vi "crio_FPGA_Antagonist_Radial.vi"() -> ()   [LabVIEW 2019]
uses:
  <vilib>/rvi/Analysis/control/PID/Typedef/niFpgaPID_ManualControl.ctl
  <vilib>/rvi/Analysis/control/PID/Typedef/niFpgaPID_PIGains.ctl
  <vilib>/rvi/Analysis/control/PID/Typedef/niFpgaPID_OutputRange.ctl
  <vilib>/rvi/Emulation/niFpgaSctlEmulationGetInTimedLoop.vi
  <vilib>/rvi/Emulation/niFpgaProcessEmulError.vi
  <vilib>/rvi/eio/common/nirviEmuTemplateMethod_errors.vi
  <vilib>/rvi/Emulation/niFpgaGetClockAttributes.vi
  <vilib>/rvi/Emulation/niFpgaEmulationReportErrorSimple.vi
  <vilib>/rvi/Emulation/niFpgaCriticalErrorInLSC.vi
  <vilib>/rvi/Analysis/control/PID/SubVIs/niFpgaPID_PIWrapper.vi
  <vilib>/eio/EIOMethodNode/EIOMethodNode.xnode
  <vilib>/eio/EIONode/EIONode.xnode
panel:
  in  "LAC Lock":bool
  in  "VCA Gains":T1 {"proportional gain" step=0.125}
  in  "LAC DC PWM Period (us)":i16=50
  in  "Debug: ConnectorA/DIO15":bool
  in  "Debug: ConnectorA/DIO14":bool
  in  "Encoder Debug":bool
  in  "Loop Timer DAQ":u32=1 caption="LAC Loop Time(uSec)"
  in  "Position Reset":bool
  out "LAC Position (Counts)":i32
  out "LAC B":bool
  out "LAC A":bool
  out "LAC B'":bool
  out "LAC A'":bool
  in  "LAC Velocity Interval (uSec)":u32=1000
  out "LAC Acceleration (Counts/Interval)":i32
  out "LAC Velocity (Counts/Interval)":i32
  out "LAC Controller PWM Output":sgl
  in  "LAC Manual Control":T2 {"manual input (0)" scale=-1.0..1.0}
  in  "LAC Setpoint":i32
  in  "LAC Gains":T1 {"proportional gain" step=0.125}
  in  "stop 2":bool
  in  "rail Initial Position":i16=1
  out "rail Platform Position":i16
  in  "Stepper Direction":bool
  in  "Stepper Enable":bool
  in  "Position Control: Desired Positoin":i16=100
  in  "Manual Operation":bool
  out "Controller Enable":bool
  out "Controller Direction":bool
  in  "mSec to initialize a small push away from limit switch":u32=1 caption="mSec when hit limit"
  in  "mSec when hit limit":u32=100 caption="rail mSec to pause when hit limit"
  in  "Rail soft limit":i16=10000
  out "Limit Switch":bool
  in  "Half Peirod (pulse 40MHz)":u32=10000 caption="rail Count(Tick) [Interval between step]"
  out "VCA ControllerPWM Output":sgl
  in  "VCA Manual Control":T2 {"manual input (0)" scale=-1.0..1.0}
  in  "VCA Position Setpoint":i32
  in  "Loop Timer DAQ 2":u32=1 caption="Loop Time(uSec)"
  in  "VCA Position Reset":bool
  out "Position (Counts) VCA":i32=-5
  out "B VCA":bool
  out "A VCA":bool=TRUE
  out "B' VCA":bool
  out "A' VCA":bool=TRUE
  in  "Velocity Interval (uSec)":u32=1000
  out "Acceleration (Counts/Interval) VCA":i32
  out "Velocity (Counts/Interval) VCA":i32
  in  "DC PWM Period (microsec)":i16=50
  in  "stop":bool=TRUE
  # "Period Default 500(us) 2kHz"
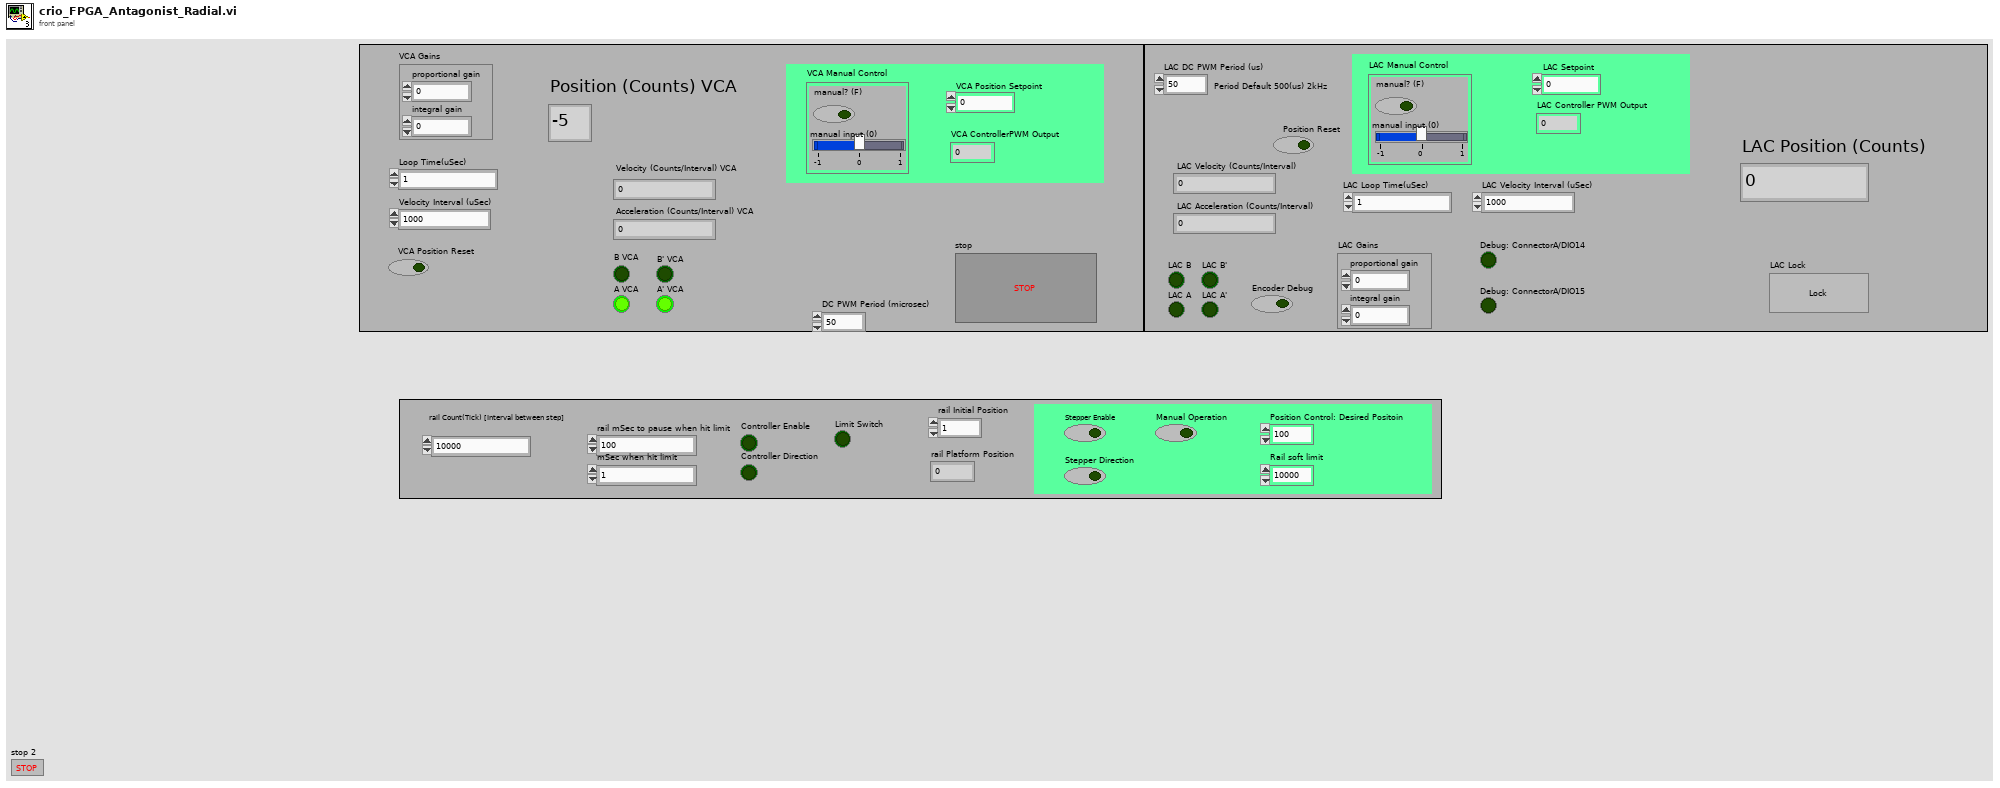
[diagram p1: front panel]
types:
  T1 = typedef "niFpgaPID_PIGains.ctl" = cluster{"proportional gain":sgl, "integral gain":sgl}
  T2 = typedef "niFpgaPID_ManualControl.ctl" = cluster{"manual? (F)":bool, "manual input (0)":sgl}
  T3 = typedef "niFpgaPID_OutputRange.ctl" = cluster{"output high (Inf)":sgl, "output low (-Inf)":sgl}
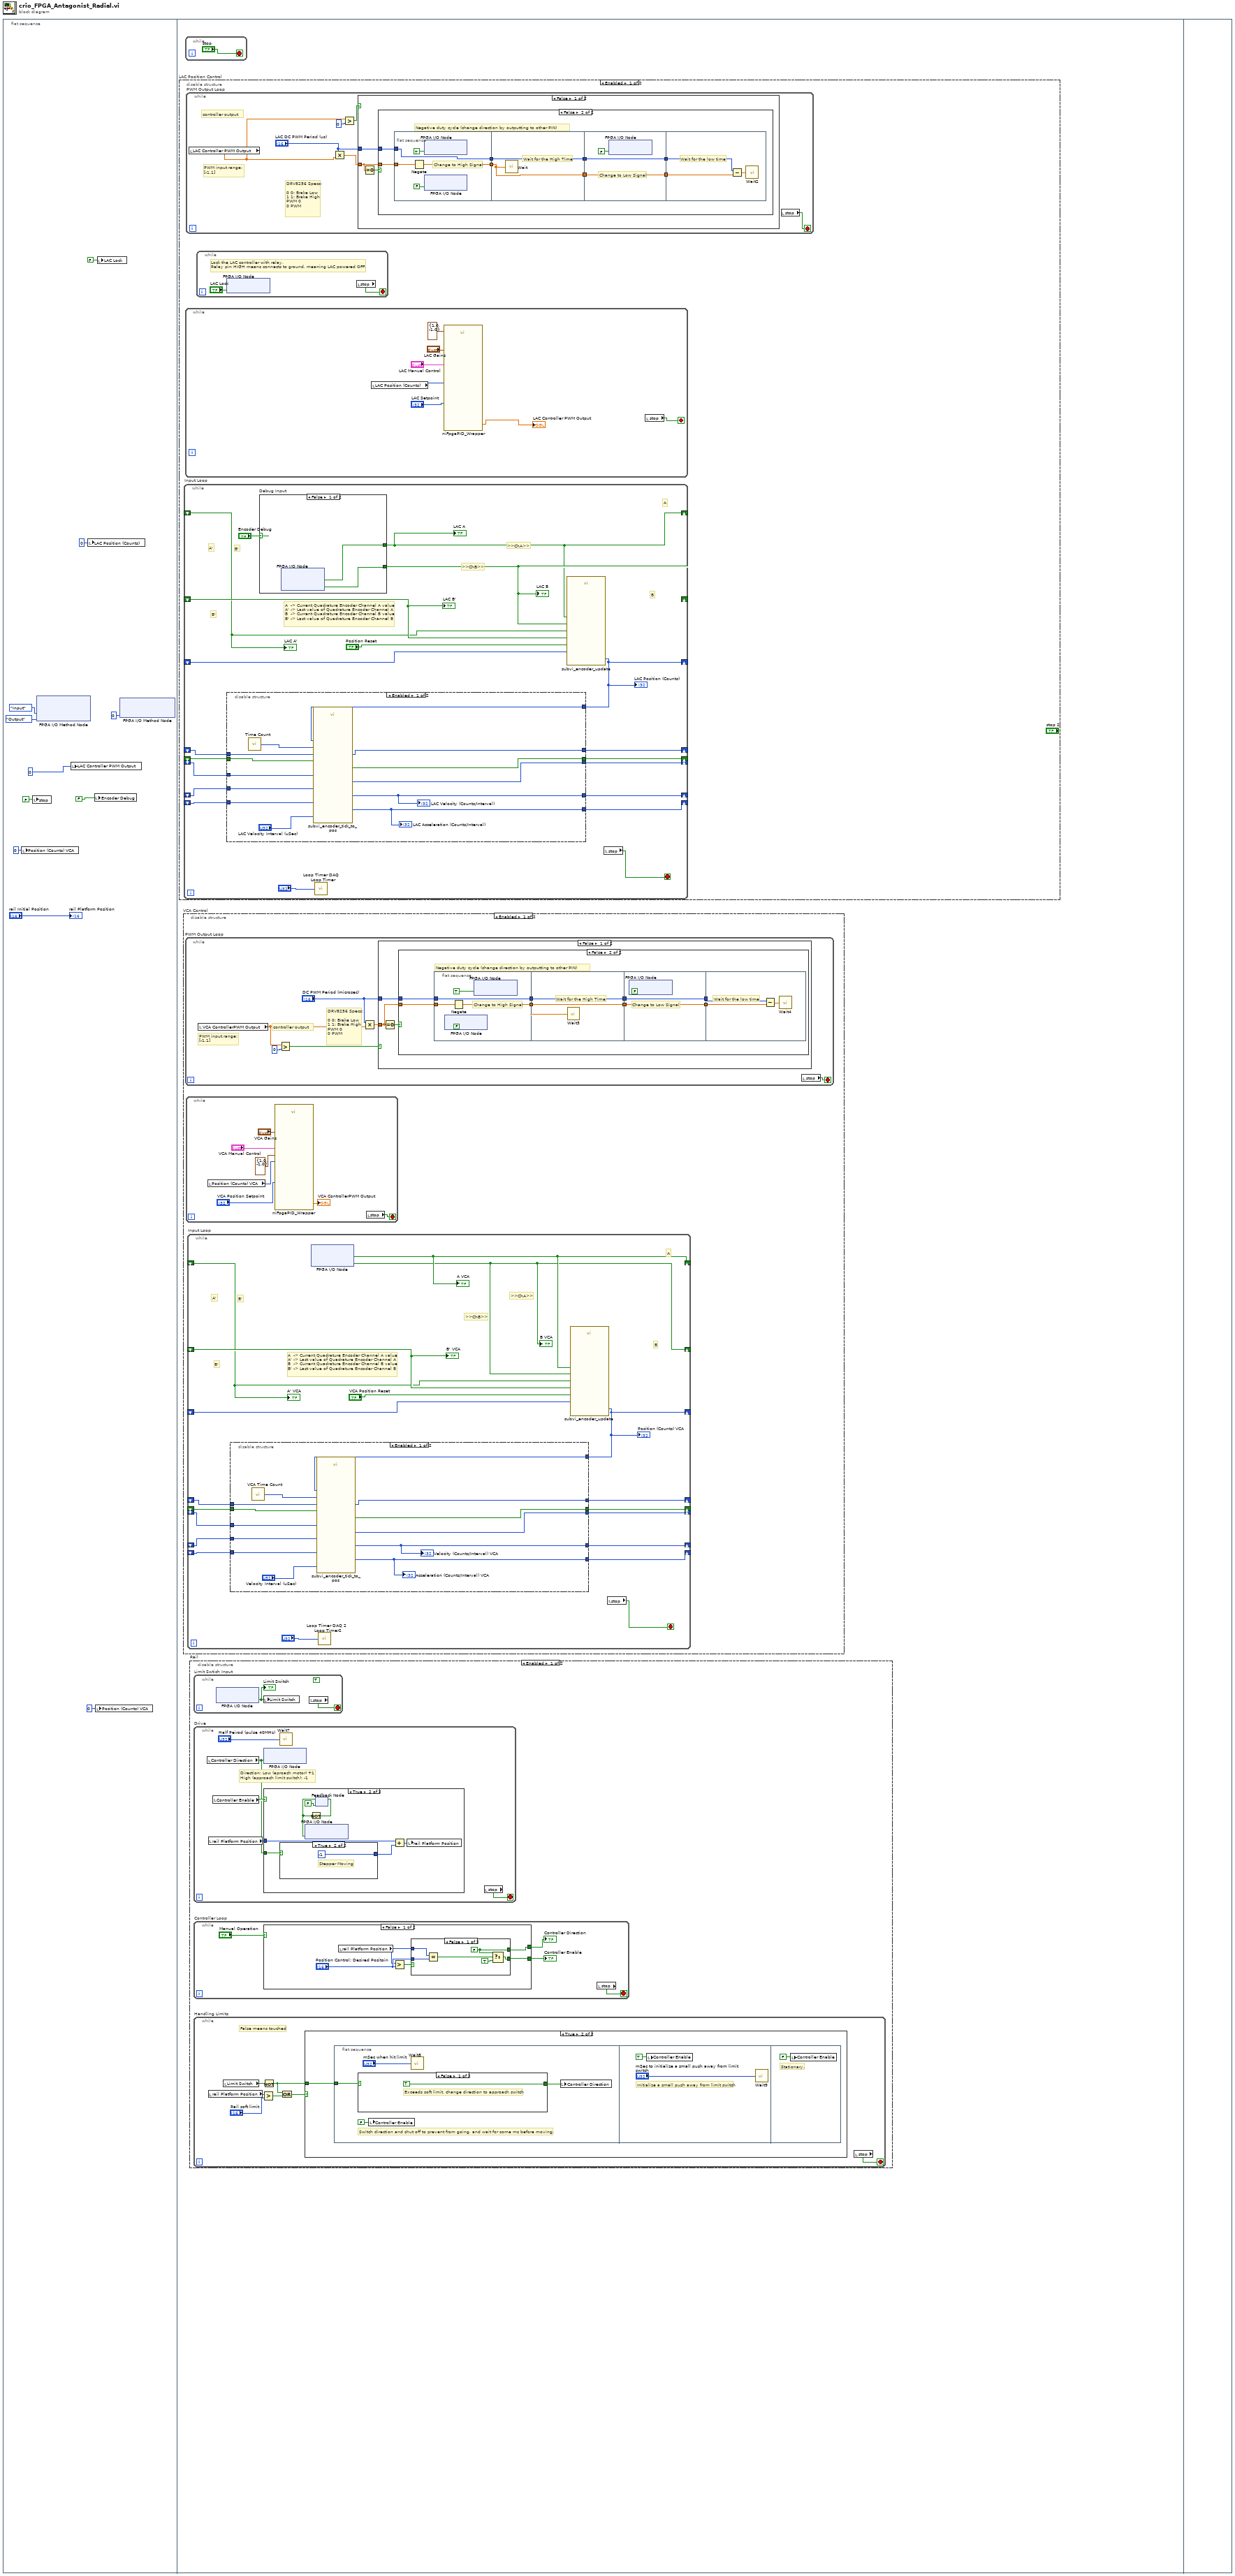
[diagram p0: block diagram]
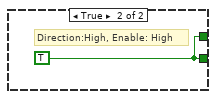
[diagram p2: hidden frame]
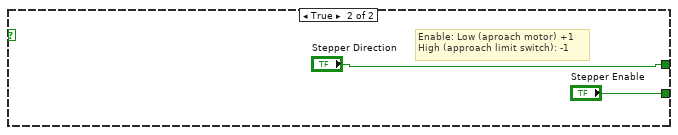
[diagram p3: hidden frame]
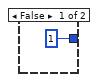
[diagram p5: hidden frame]
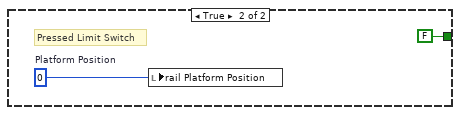
[diagram p7: hidden frame]
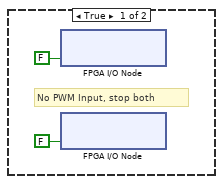
[diagram p10: hidden frame]
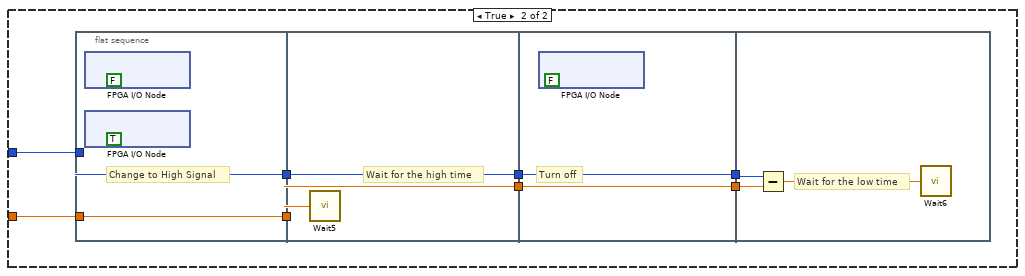
[diagram p11: hidden frame]
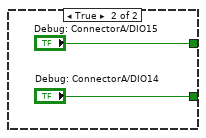
[diagram p14: hidden frame]
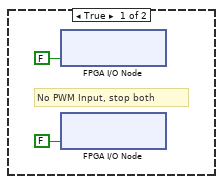
[diagram p15: hidden frame]
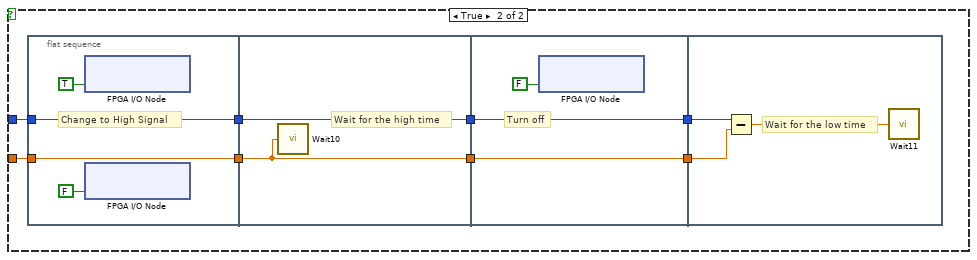
[diagram p16: hidden frame]
diagram:
  n1 = flat-sequence {
    frame #0 {
      n2 = local write "Position (Counts) VCA"(0 ("LAC Position (Counts)")) -> ()
      n3 = local write "stop"(FALSE ("stop")) -> ()
      n4 = xnode "FPGA I/O Method Node"("DIO 7:4"=enum8{"No Change", "Input", "Output"}."Input", "DIO 3:0"=enum8{"No Change", "Input", "Output"}."Output") -> ()  [unwired: 1 in, 1 out]
      n5 = local write "LAC Controller PWM Output"(u32 0 ("Servo wait time")) -> ()
      n6 = local write "LAC Position (Counts)"(0 ("LAC Position (Counts)")) -> ()
      n7 = local write "Encoder Debug"(FALSE ("LAC Lock")) -> ()
      n8 = local write "Position (Counts) VCA"(0 ("Position (Counts) VCA")) -> ()
      n9 = local write "LAC Lock"(FALSE ("LAC Lock")) -> ()
      n10 = xnode "FPGA I/O Method Node"("Enable"=u8 0) -> ()  [unwired: 1 in, 1 out]
      "rail Platform Position" <- "rail Initial Position"
    }
    frame #1 {
      n11 = disable-structure "LAC Position Control" shown="Enabled" {
        frame Enabled {
          n12 = while "Input Loop" {
            shift-right: [w178] -> _
            shift-left: _ -> [w181]
            shift-right: [w177] -> _
            shift-left: _ -> [w180]
            shift-right: [w173] -> _
            shift-left: _ -> [w179]
            shift-right: [w166] -> _
            shift-left: _ -> [w176]
            shift-right: [w167] -> _
            shift-left: _ -> [w175]
            shift-right: [w174] -> _
            shift-left: _ -> [w172]
            shift-right: [w171] -> _
            shift-left: _ -> [w170]
            shift-right: [w169] -> _
            shift-left: _ -> [w168]
            stop <- w165 stop-if-true
            # "B'"
            # ">>ChB>>"
            # ">>ChA>>"
            # "A'"
            # "A  -> Current Quadrature Encoder Channel A value\nA' -> Last value of Quadrature Encoder Channel A\nB  -> Current Quadrature Encoder Channel B value\nB' -> Last value of Quadrature Encoder Channel B"
            # "B'"
            # "B"
            # "A"
            n13 = case "Debug Input" shown="False" "Encoder Debug" {
              tunnel: [w199 "Debug: ConnectorA/DIO15"] -> w177
              tunnel: [w198 "Debug: ConnectorA/DIO14"] -> w178
              frame False {
                n14 = xnode "FPGA I/O Node"() -> ("Mod2/DIO2"=w199:bool, "Mod2/DIO3"=w198:bool)  [unwired: 2 in, 2 out]
              }
              frame True {
              }
            }
            "LAC B" <- w178
            "LAC A" <- w177
            n15 = call "Loop Timer"("Count(uSec)"="Loop Timer DAQ") -> ()  [unwired: 1 out]
            n16 = call "subvi_encoder_update.vi"("Position Reset"="Position Reset", "Tick'"=w179, "A"=w177, "B'"=w181, "A'"=w180, "B"=w178) -> ("Tick"=w173:i32)  [unwired: 5 in]
            "LAC Position (Counts)" <- w173
            n17 = disable-structure shown="Enabled" {
              disable-tunnel: w176 -> [w196 _]
              disable-tunnel: w175 -> [w195 _]
              disable-tunnel: [w194 _] -> w174
              disable-tunnel: w173 -> [w193 _]
              disable-tunnel: w172 -> [w192 _]
              disable-tunnel: [w191 _] -> w171
              disable-tunnel: w170 -> [w190 _]
              disable-tunnel: [w189 _] -> w169
              disable-tunnel: w168 -> [w188 _]
              disable-tunnel: [w186 _] -> w167
              disable-tunnel: [w185 _] -> w166
              frame Enabled {
                n18 = call "Time Count"() -> ("Tick Count(uSec)"=w187:u32)
                n19 = call "subvi_encoder_tick_to_pos.vi"("Velocity Interval (uSec)"="LAC Velocity Interval (uSec)", "Raw Tick"=w193, "Waited?'"=w190, "Tick Count(uSec)'"=w188, "p'"=w192, "Time Count"=w187, "a'"=w195, "v'"=w196) -> ("Waited?"=w191:bool, "Tick Count(uSec)"=w189:u32, "p"=w194:i32, "a"=w186:i32, "v"=w185:i32)  [unwired: 3 in]
                "LAC Acceleration (Counts/Interval)" <- w186
                "LAC Velocity (Counts/Interval)" <- w185
              }
              frame Disabled {
              }
            }
            n20 = local read "stop"() -> (w165:bool)
            "LAC B'" <- w181
            "LAC A'" <- w180
          }
          n21 = while {
            stop <- w164 stop-if-true
            n22 = local read "LAC Position (Counts)"() -> (w163:i32)
            n23 = call-poly <vilib>:"niFpgaPID_Wrapper.vi"("setpoint"="LAC Setpoint", "process variable"=w163, "manual control"="LAC Manual Control", "gains"="LAC Gains", "output range"=T3 {"output high (Inf)"=1.0, "output low (-Inf)"=-1.0}) -> ("output"=→"LAC Controller PWM Output":sgl)  [unwired: 8 in, 2 out]
            n24 = local read "stop"() -> (w164:bool)
          }
          n25 = while "PWM Output Loop" {
            stop <- w202 stop-if-true
            # "PWM input range:\n[-1,1]"
            # "DRV8256 Specs:\n\n0 0: Brake Low\n1 1: Brake High\nPWM 0\n0 PWM"
            # "controller output"
            n26 = local read "LAC Controller PWM Output"() -> (w203:sgl)
            n27 = Multiply(x="LAC DC PWM Period (us)", y=w203) -> (x*y=w205:sgl)
            n28 = Greater?(x=w203, y=i16 0) -> (0:w206:bool)
            n29 = case shown="False" w206 {
              tunnel: w205 -> [w210 w241]
              tunnel: "LAC DC PWM Period (us)" -> [w208 w240]
              frame False {
                n30 = Equal To 0?(x=w210) -> (x = 0?=w209:bool)
                n31 = case shown="False" w209 {
                  tunnel: w210 -> [_ w220]
                  tunnel: w208 -> [_ w213]
                  frame True {
                    # "No PWM Input, stop both"
                    n32 = xnode "FPGA I/O Node"("Mod1/DIO2"=FALSE) -> ()  [unwired: 1 in, 1 out]
                    n33 = xnode "FPGA I/O Node"("Mod1/DIO3"=FALSE) -> ()  [unwired: 1 in, 1 out]
                  }
                  frame False {
                    # "Negative duty cycle (change direction by outputting to other PIN)"
                    n34 = flat-sequence {
                      tunnel: w220 -> [w223]
                      tunnel: [w222] -> w219
                      tunnel: [w221] -> w214
                      tunnel: w213 -> [w221]
                      tunnel: w219 -> [w227]
                      tunnel: [w227] -> w218
                      tunnel: [w226] -> w215
                      tunnel: w214 -> [w226]
                      tunnel: w218 -> [w229]
                      tunnel: [w229] -> w217
                      tunnel: [w228] -> w216
                      tunnel: w215 -> [w228]
                      tunnel: w217 -> [w233]
                      tunnel: w216 -> [w232]
                      frame #0 {
                        # "Change to High Signal"
                        n35 = Negate(x=w223) -> (-x=w222:sgl)
                        n36 = xnode "FPGA I/O Node"("Mod1/DIO3"=TRUE) -> ()  [unwired: 1 in, 1 out]
                        n37 = xnode "FPGA I/O Node"("Mod1/DIO2"=FALSE) -> ()  [unwired: 1 in, 1 out]
                      }
                      frame #1 {
                        # "Wait for the High Time"
                        n38 = call "Wait"("Count(uSec)"=w227) -> ()  [unwired: 1 out]
                      }
                      frame #2 {
                        # "Change to Low Signal"
                        n39 = xnode "FPGA I/O Node"("Mod1/DIO2"=FALSE) -> ()  [unwired: 1 in, 1 out]
                      }
                      frame #3 {
                        # "Wait for the low time"
                        n40 = Subtract(x=w232, y=w233) -> (x-y=w231:sgl)
                        n41 = call "Wait2"("Count(uSec)"=w231) -> ()  [unwired: 1 out]
                      }
                    }
                  }
                }
              }
              frame True {
                n42 = flat-sequence {
                  tunnel: w241 -> [w242]
                  tunnel: w240 -> [w243]
                  tunnel: [w243] -> w237
                  tunnel: [w242] -> w236
                  tunnel: [w247] -> w238
                  tunnel: w237 -> [w247]
                  tunnel: w236 -> [w246]
                  tunnel: [w246] -> w235
                  tunnel: [w249] -> w239
                  tunnel: w238 -> [w249]
                  tunnel: w235 -> [w248]
                  tunnel: [w248] -> w234
                  tunnel: w239 -> [w253]
                  tunnel: w234 -> [w251]
                  frame #0 {
                    # "Change to High Signal"
                    n43 = xnode "FPGA I/O Node"("Mod1/DIO2"=TRUE) -> ()  [unwired: 1 in, 1 out]
                    n44 = xnode "FPGA I/O Node"("Mod1/DIO3"=FALSE ("ConnectorB/DIO9")) -> ()  [unwired: 1 in, 1 out]
                  }
                  frame #1 {
                    # "Wait for the high time"
                    n45 = call "Wait10"("Count(uSec)"=w246) -> ()  [unwired: 1 out]
                  }
                  frame #2 {
                    # "Turn off"
                    n46 = xnode "FPGA I/O Node"("Mod1/DIO2"=FALSE) -> ()  [unwired: 1 in, 1 out]
                  }
                  frame #3 {
                    # "Wait for the low time"
                    n47 = Subtract(x=w253, y=w251) -> (x-y=w252:sgl)
                    n48 = call "Wait11"("Count(uSec)"=w252) -> ()  [unwired: 1 out]
                  }
                }
              }
            }
            n49 = local read "stop"() -> (w202:bool)
          }
          n50 = while {
            stop <- w157 stop-if-true
            # "Lock the LAC controller with relay.\nRelay pin HIGH means connects to ground, meaning LAC powered OFF."
            n51 = xnode "FPGA I/O Node"("Mod8/DIO6"="LAC Lock") -> ()  [unwired: 1 in, 1 out]
            n52 = local read "stop"() -> (w157:bool)
          }
        }
        frame Disabled {
        }
      }
      n53 = disable-structure "VCA Control" shown="Enabled" {
        frame Enabled {
          n54 = while "PWM Output Loop" {
            stop <- w104 stop-if-true
            # "PWM input range:\n[-1,1]"
            # "DRV8256 Specs:\n\n0 0: Brake Low\n1 1: Brake High\nPWM 0\n0 PWM"
            # "controller output"
            n55 = local read "VCA ControllerPWM Output"() -> (w105:sgl)
            n56 = Greater?(x=w105, y=i16 0) -> (0:w108:bool)
            n57 = Multiply(x="DC PWM Period (microsec)", y=w105) -> (x*y=w107:sgl)
            n58 = case shown="False" w108 {
              tunnel: w107 -> [w112 w143]
              tunnel: "DC PWM Period (microsec)" -> [w110 w142]
              frame False {
                n59 = Equal To 0?(x=w112) -> (x = 0?=w111:bool)
                n60 = case shown="False" w111 {
                  tunnel: w112 -> [_ w122]
                  tunnel: w110 -> [_ w115]
                  frame True {
                    # "No PWM Input, stop both"
                    n61 = xnode "FPGA I/O Node"("Mod1/DIO1"=FALSE) -> ()  [unwired: 1 in, 1 out]
                    n62 = xnode "FPGA I/O Node"("Mod1/DIO0"=FALSE) -> ()  [unwired: 1 in, 1 out]
                  }
                  frame False {
                    # "Negative duty cycle (change direction by outputting to other PIN)"
                    n63 = flat-sequence {
                      tunnel: w122 -> [w125]
                      tunnel: [w124] -> w121
                      tunnel: [w123] -> w116
                      tunnel: w115 -> [w123]
                      tunnel: w121 -> [w129]
                      tunnel: [w129] -> w120
                      tunnel: [w128] -> w117
                      tunnel: w116 -> [w128]
                      tunnel: w120 -> [w131]
                      tunnel: [w131] -> w119
                      tunnel: [w130] -> w118
                      tunnel: w117 -> [w130]
                      tunnel: w119 -> [w135]
                      tunnel: w118 -> [w134]
                      frame #0 {
                        # "Change to High Signal"
                        n64 = xnode "FPGA I/O Node"("Mod1/DIO0"=FALSE) -> ()  [unwired: 1 in, 1 out]
                        n65 = Negate(x=w125) -> (-x=w124:sgl)
                        n66 = xnode "FPGA I/O Node"("Mod1/DIO1"=TRUE) -> ()  [unwired: 1 in, 1 out]
                      }
                      frame #1 {
                        # "Wait for the High Time"
                        n67 = call "Wait3"("Count(uSec)"=w129) -> ()  [unwired: 1 out]
                      }
                      frame #2 {
                        # "Change to Low Signal"
                        n68 = xnode "FPGA I/O Node"("Mod1/DIO1"=FALSE) -> ()  [unwired: 1 in, 1 out]
                      }
                      frame #3 {
                        # "Wait for the low time"
                        n69 = Subtract(x=w134, y=w135) -> (x-y=w133:sgl)
                        n70 = call "Wait4"("Count(uSec)"=w133) -> ()  [unwired: 1 out]
                      }
                    }
                  }
                }
              }
              frame True {
                n71 = flat-sequence {
                  tunnel: w143 -> [w144]
                  tunnel: w142 -> [w145]
                  tunnel: [w145] -> w139
                  tunnel: [w144] -> w138
                  tunnel: [w149] -> w140
                  tunnel: w139 -> [w149]
                  tunnel: w138 -> [w148]
                  tunnel: [w148] -> w137
                  tunnel: [w151] -> w141
                  tunnel: w140 -> [w151]
                  tunnel: w137 -> [w150]
                  tunnel: [w150] -> w136
                  tunnel: w141 -> [w155]
                  tunnel: w136 -> [w153]
                  frame #0 {
                    # "Change to High Signal"
                    n72 = xnode "FPGA I/O Node"("Mod1/DIO1"=FALSE ("ConnectorB/DIO9")) -> ()  [unwired: 1 in, 1 out]
                    n73 = xnode "FPGA I/O Node"("Mod1/DIO0"=TRUE) -> ()  [unwired: 1 in, 1 out]
                  }
                  frame #1 {
                    # "Wait for the high time"
                    n74 = call "Wait5"("Count(uSec)"=w148) -> ()  [unwired: 1 out]
                  }
                  frame #2 {
                    # "Turn off"
                    n75 = xnode "FPGA I/O Node"("Mod1/DIO0"=FALSE) -> ()  [unwired: 1 in, 1 out]
                  }
                  frame #3 {
                    # "Wait for the low time"
                    n76 = Subtract(x=w155, y=w153) -> (x-y=w154:sgl)
                    n77 = call "Wait6"("Count(uSec)"=w154) -> ()  [unwired: 1 out]
                  }
                }
              }
            }
            n78 = local read "stop"() -> (w104:bool)
          }
          n79 = while {
            stop <- w103 stop-if-true
            n80 = local read "Position (Counts) VCA"() -> (w102:i32)
            n81 = call-poly <vilib>:"niFpgaPID_Wrapper.vi"("setpoint"="VCA Position Setpoint", "process variable"=w102, "manual control"="VCA Manual Control", "gains"="VCA Gains", "output range"=T3 {"output high (Inf)"=1.0, "output low (-Inf)"=-1.0}) -> ("output"=→"VCA ControllerPWM Output":sgl)  [unwired: 8 in, 2 out]
            n82 = local read "stop"() -> (w103:bool)
          }
          n83 = while "Input Loop" {
            shift-right: [w65] -> _
            shift-left: _ -> [w81]
            shift-right: [w66] -> _
            shift-left: _ -> [w80]
            shift-right: [w75] -> _
            shift-left: _ -> [w79]
            shift-right: [w68] -> _
            shift-left: _ -> [w78]
            shift-right: [w69] -> _
            shift-left: _ -> [w77]
            shift-right: [w76] -> _
            shift-left: _ -> [w74]
            shift-right: [w73] -> _
            shift-left: _ -> [w72]
            shift-right: [w71] -> _
            shift-left: _ -> [w70]
            stop <- w67 stop-if-true
            # "B'"
            # ">>ChB>>"
            # ">>ChA>>"
            # "A'"
            # "A  -> Current Quadrature Encoder Channel A value\nA' -> Last value of Quadrature Encoder Channel A\nB  -> Current Quadrature Encoder Channel B value\nB' -> Last value of Quadrature Encoder Channel B"
            # "B'"
            # "B"
            # "A"
            n84 = xnode "FPGA I/O Node"() -> ("Mod2/DIO0"=w66:bool, "Mod2/DIO1"=w65:bool)  [unwired: 2 in, 2 out]
            "B VCA" <- w65
            "A VCA" <- w66
            n85 = call "Loop Timer2"("Count(uSec)"="Loop Timer DAQ 2") -> ()  [unwired: 1 out]
            n86 = call "subvi_encoder_update.vi"("Position Reset"="VCA Position Reset", "Tick'"=w79, "A"=w66, "B'"=w81, "A'"=w80, "B"=w65) -> ("Tick"=w75:i32)  [unwired: 5 in]
            "Position (Counts) VCA" <- w75
            n87 = disable-structure shown="Enabled" {
              disable-tunnel: w78 -> [w95 _]
              disable-tunnel: w77 -> [w94 _]
              disable-tunnel: [w93 _] -> w76
              disable-tunnel: w75 -> [w92 _]
              disable-tunnel: w74 -> [w91 _]
              disable-tunnel: [w90 _] -> w73
              disable-tunnel: w72 -> [w89 _]
              disable-tunnel: [w88 _] -> w71
              disable-tunnel: w70 -> [w87 _]
              disable-tunnel: [w85 _] -> w69
              disable-tunnel: [w84 _] -> w68
              frame Enabled {
                n88 = call "VCA Time Count"() -> ("Tick Count(uSec)"=w86:u32)
                n89 = call "subvi_encoder_tick_to_pos.vi"("Velocity Interval (uSec)"="Velocity Interval (uSec)", "Raw Tick"=w92, "Waited?'"=w89, "Tick Count(uSec)'"=w87, "p'"=w91, "Time Count"=w86, "a'"=w94, "v'"=w95) -> ("Waited?"=w90:bool, "Tick Count(uSec)"=w88:u32, "p"=w93:i32, "a"=w85:i32, "v"=w84:i32)  [unwired: 3 in]
                "Acceleration (Counts/Interval) VCA" <- w85
                "Velocity (Counts/Interval) VCA" <- w84
              }
              frame Disabled {
              }
            }
            n90 = local read "stop"() -> (w67:bool)
            "B' VCA" <- w81
            "A' VCA" <- w80
          }
        }
        frame Disabled {
        }
      }
      n91 = while {
        stop <- "stop" stop-if-true
      }
      n92 = disable-structure "Rail" shown="Enabled" {
        frame Enabled {
          n93 = while "Limit Swtich Input" {
            stop <- w63 stop-if-true
            (unwired) TRUE ("Mod8/DIO2")
            n94 = xnode "FPGA I/O Node"() -> ("Mod8/DIO2"=w64:bool)  [unwired: 1 in, 1 out]
            "Limit Switch" <- w64
            n95 = local write "Limit Switch"(w64) -> ()
            n96 = local read "stop"() -> (w63:bool)
          }
          n97 = while "Drive" {
            stop <- w31 stop-if-true
            # "Direction: Low (aproach motor) +1\nHigh (approach limit switch): -1"
            n98 = local read "Controller Direction"() -> (w32:bool)
            n99 = local read "rail Platform Position"() -> (w34:i16)
            n100 = local read "Controller Enable"() -> (w33:bool)
            n101 = xnode "FPGA I/O Node"("Mod8/DIO4"=w32) -> ()  [unwired: 1 in, 1 out]
            n102 = case shown="True" w33 {
              tunnel: w32 -> [_ w39]
              tunnel: w34 -> [_ w36]
              frame False {
              }
              frame True {
                n103 = case shown="True" w39 {
                  tunnel: [i16 1 i16 -1] -> w38
                  frame False {
                  }
                  frame True {
                    # "Stepper Moving"
                  }
                }
                n104 = feedback #1(FALSE ("Connector0/DIO0")) -> (w40:bool)
                n105 = xnode "FPGA I/O Node"("Mod8/DIO3"=w40) -> ()  [unwired: 1 in, 1 out]
                n106 = Not(x=w40) -> (.not. x?=w41:bool)
                n107 = feedback-in #1(w41) -> ()
                n108 = Add(x=w36, y=w38) -> (x+y=w37:i16)
                n109 = local write "rail Platform Position"(w37) -> ()
              }
            }
            n110 = call "Wait7"("Count(Ticks)"="Half Peirod (pulse 40MHz)") -> ()  [unwired: 1 out]
            n111 = local read "stop"() -> (w31:bool)
          }
          n112 = while "Controller Loop" {
            stop <- w16 stop-if-true
            n113 = case shown="False" "Manual Operation" {
              tunnel: [w20 "Stepper Enable"] -> w14
              tunnel: [w19 "Stepper Direction"] -> w13
              frame False {
                n114 = local read "rail Platform Position"() -> (w17:i16)
                n115 = Greater?(x=w17, y="Position Control: Desired Positoin") -> (0:w21:bool)
                n116 = case shown="False" w21 {
                  tunnel: [w24 w28] -> w20
                  tunnel: [w22 w28] -> w19
                  tunnel: "Position Control: Desired Positoin" -> [w27 _]
                  tunnel: w17 -> [w26 _]
                  frame False {
                    w22 = FALSE
                    n117 = Equal?(x=w26, y=w27) -> (x = y?=w25:bool)
                    n118 = Select(t=w22, s=w25, f=TRUE) -> (s? t:f=w24:bool)
                  }
                  frame True {
                    w28 = TRUE
                    # "Direction:High, Enable: High"
                  }
                }
              }
              frame True {
                # "Enable: Low (aproach motor) +1\nHigh (approach limit switch): -1"
              }
            }
            "Controller Enable" <- w14
            "Controller Direction" <- w13
            n119 = local read "stop"() -> (w16:bool)
          }
          n120 = while "Handling Limits" {
            stop <- w51 stop-if-true
            # "False means touched"
            n121 = local read "rail Platform Position"() -> (w50:i16)
            n122 = local read "Limit Switch"() -> (w46:bool)
            n123 = Greater?(x=w50, y="Rail soft limit") -> (0:w48:bool)
            n124 = Not(x=w46) -> (.not. x?=w45:bool)
            n125 = Or(x=w45, y=w48) -> (x .or. y?=w47:bool)
            n126 = case shown="True" w47 {
              tunnel: w45 -> [_ w52]
              frame False {
                # "Do nothing"
              }
              frame True {
                n127 = flat-sequence {
                  tunnel: w52 -> [w53]
                  frame #0 {
                    # "Switch direction and shut off to prevent from going, and wait for some ms before moving."
                    n128 = case shown="False" w53 {
                      tunnel: [TRUE ("Stepper Direction") FALSE ("Stepper Direction")] -> w54
                      frame False {
                        # "Exceeds soft limit, change direction to approach switch"
                      }
                      frame True {
                        w59 = i16 0  # Platform Position
                        # "Pressed Limit Switch"
                        n129 = local write "rail Platform Position"(w59) -> ()
                      }
                    }
                    n130 = local write "Controller Enable"(FALSE ("Stepper Direction")) -> ()
                    n131 = call "Wait8"("Count(mSec)"="mSec when hit limit") -> ()  [unwired: 1 out]
                    n132 = local write "Controller Direction"(w54) -> ()
                  }
                  frame #1 {
                    # "Initialize a small push away from limit switch"
                    n133 = local write "Controller Enable"(TRUE ("Stepper Enable")) -> ()
                    n134 = call "Wait9"("Count(mSec)"="mSec to initialize a small push away from limit switch") -> ()  [unwired: 1 out]
                  }
                  frame #2 {
                    # "Stationary."
                    n135 = local write "Controller Enable"(FALSE ("Stepper Enable")) -> ()
                  }
                }
              }
            }
            n136 = local read "stop"() -> (w51:bool)
          }
        }
        frame Disabled {
        }
      }
    }
    frame #2 {
    }
  }
